vi "Change_image_properties.vi"(8 "error in (no error)":errorcluster, 11 "Path In":path) -> (0 "error out":errorcluster, 3 "Path Out":path)   [LabVIEW 2016]
uses:
  <vilib>/vision/NI_Vision_Development_Module.lvlib
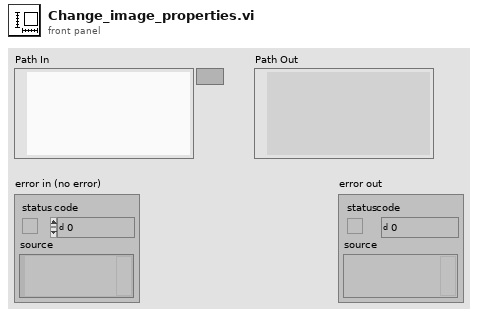
[diagram p1: front panel]
types:
  T1 = typedef "IMAQ Image.ctl" = refnum<image>
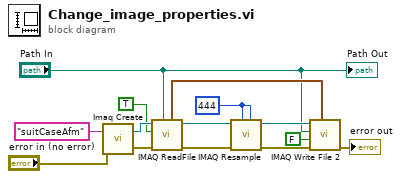
[diagram p0: block diagram]
diagram:
  w10 = 444 ("Y Resolution")
  n1 = call "Imaq Create"("Image Name"="suitCaseAfm", "error in (no error)"="error in (no error)") -> ("New Image"=w9:T1, "error out"=w8:errorcluster)  [unwired: 3 in]
  n2 = call "IMAQ ReadFile"("File Path"="Path In", "error in (no error)"=w8, "Load Color Palette? (No)"=TRUE, "Image"=w9) -> ("error out"=w13:errorcluster, "Image Out"=w14:T1, "Color Palette out"=w5:cluster{"Red":u8, "Green":u8, "Blue":u8}[])  [unwired: 3 in, 2 out]
  n3 = call "IMAQ Resample"("X Resolution"=w10, "Y Resolution"=w10, "error in (no error)"=w13, "Image Src"=w14) -> ("error out"=w11:errorcluster, "Image Dst Out"=w12:T1)  [unwired: 6 in]
  n4 = call-poly "IMAQ Write File 2"("Color Palette"=w5, "error in (no error)"=w11, "Compress? (N)"=FALSE, "File Path"="Path In", "Image"=w12) -> ("error out"=→"error out":errorcluster)  [unwired: 5 in, 1 out]
  "Path Out" <- "Path In"
